vi "InitFT.vi"(3 "Timing parameters":T1={"Sample Rate"=1000.0, "Samples to Read"=100}, 4 "Transform":T4, 5 "Channel Parameters":T2={"First Channel"=1, "Number of Channels"=6, "DAQ Card"="Dev2", "Maximum Value"=10.0, "Minimum Value"=-10.0}, 6 "Sensor Parameters":T3={"Calibration File"=path "D:/ArduinoSmarticle/entangledSmarticle/FT21164.cal", "Force Units"="N", "Torque Units"="N-mm"}) -> (0 "error out":errorcluster, 1 "task out":refnum<k21>, 2 "Calibration Matrix":dbl[][](array[numeric]))   [LabVIEW 2012]
uses:
  <vilib>/DAQmx/create/channels.llb/DAQmx Create Channel (AI-Voltage-Basic).vi
  <vilib>/DAQmx/configure/timing.llb/DAQmx Timing (Sample Clock).vi
panel:
  out "Force Units":string
  out "Torque Units":string
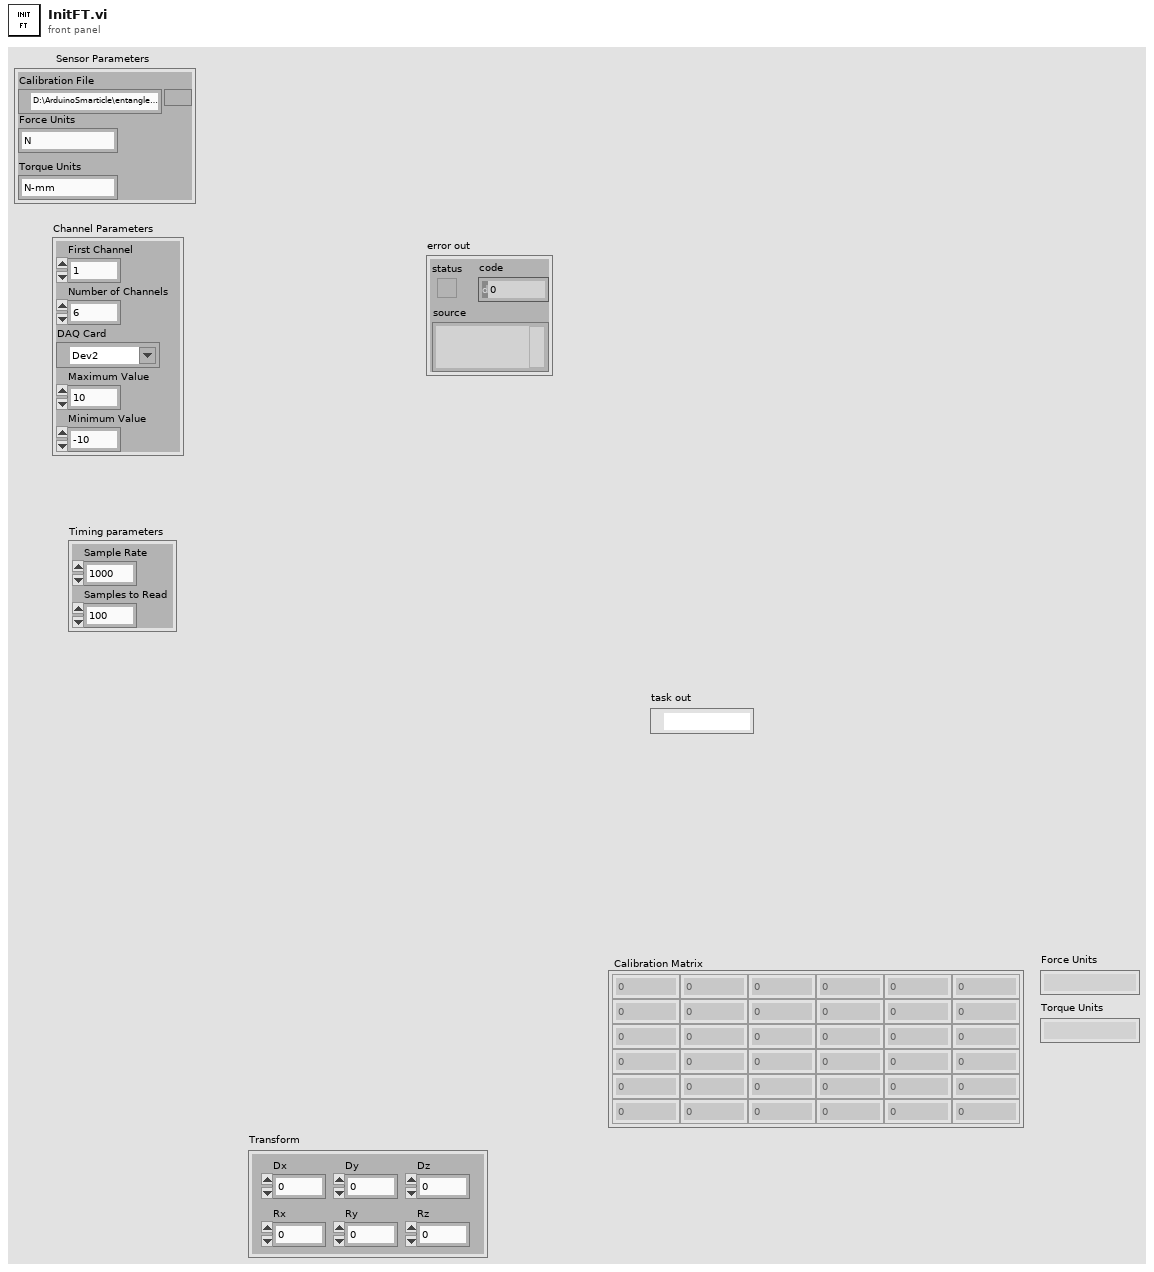
[diagram p1: front panel]
types:
  T1 = cluster{"Sample Rate":dbl, "Samples to Read":i32}
  T2 = cluster{"First Channel":i16, "Number of Channels":i16, "DAQ Card":tag, "Maximum Value":dbl, "Minimum Value":dbl}
  T3 = cluster{"Calibration File":path, "Force Units":string, "Torque Units":string}
  T4 = cluster{"Dx":dbl, "Dy":dbl, "Dz":dbl, "Rx":dbl, "Ry":dbl, "Rz":dbl}
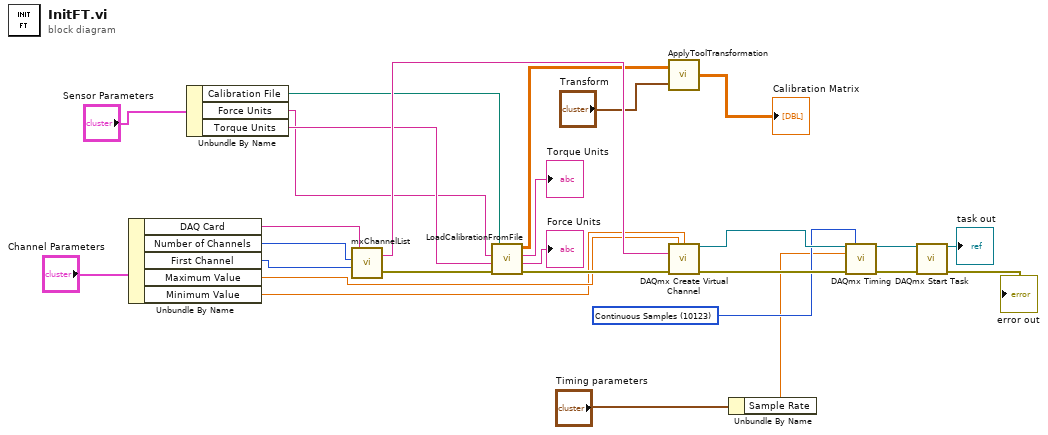
[diagram p0: block diagram]
diagram:
  w25 = 10123 items=["Finite Samples"=10178, "Continuous Samples"=10123] ("sample mode")
  n1 = Unbundle By Name("Channel Parameters") -> ("DAQ Card"=w5:tag, "Number of Channels"=w6:i16, "First Channel"=w7:i16, "Maximum Value"=w9:dbl, "Minimum Value"=w8:dbl)
  n2 = Unbundle By Name("Sensor Parameters") -> ("Calibration File"=w11:path, "Force Units"=w12:string, "Torque Units"=w13:string)
  n3 = call "mxChannelList.vi"("First Channel"=w7, "Number of Channels"=w6, "DAQmx Device Name"=w5) -> ("error out"=w16:errorcluster, "Channel List"=w23:string)  [unwired: 1 in]
  n4 = call "LoadCalibrationFromFile.vi"("Error In"=w16, "User Torque Units"=w13, "User Force Units"=w12, "Cal File Path"=w11) -> ("Error Out"=w15:errorcluster, "Calibration Force Units"=→"Force Units":string, "Calibration Torque Units"=→"Torque Units":string, "Calibration Matrix"=w20:dbl[][])
  n5 = call "ApplyToolTransformation.vi"("Transform"="Transform", "Calibration Matrix"=w20) -> ("Transformed Calibration Matrix"=→"Calibration Matrix":dbl[][])
  n6 = call-poly <vilib>:"DAQmx Create Virtual Channel.vi"("maximum value"=w9, "minimum value"=w8, "physical channels"=w23, "error in"=w15) -> ("task out"=w26:refnum<k21>, "error out"=w27:errorcluster)  [unwired: 10 in]
  n7 = Unbundle By Name("Timing parameters") -> ("Sample Rate"=w4:dbl)
  n8 = call-poly <vilib>:"DAQmx Timing.vi"("task/channels in"=w26, "sample mode"=w25, "rate"=w4, "error in"=w27) -> ("task out"=w24:refnum<k21>, "error out"=w22:errorcluster)  [unwired: 10 in]
  n9 = call <vilib>:"DAQmx Start Task.vi"("task/channels in"=w24, "error in"=w22) -> ("task out"=→"task out":refnum<k21>, "error out"=→"error out":errorcluster)  [unwired: 12 in]
